vi "Unescape HTTP URL.vi"(1 "escaped string in":string) -> (0 "unescaped string out":string)   [LabVIEW 2017, in "NI_WebServices.lvlib"]
doc: "Replaces escape sequences with the corresponding special characters according to the URL encoding specification RFC 1738."
uses:
  <vilib>/wsapi/NI_WebServices.lvlib
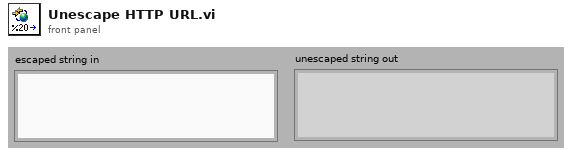
[diagram p1: front panel]
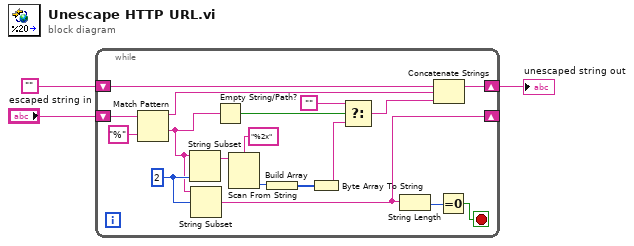
[diagram p0: block diagram]
diagram:
  n1 = while {
    shift-right: [w16] -> _
    shift-left: "escaped string in" -> [w21]
    shift-right: [w18] -> w1
    shift-left: "" -> [w17]
    stop <- w14 stop-if-true
    w19 = 2 ("length (rest)")
    n2 = Match Pattern(string=w21, regular expression="%") -> (before substring=w13:string, after substring=w4:string)  [unwired: 1 in, 2 out]
    n3 = String Subset(string=w4, length (rest)=w19) -> (substring=w10:string)  [unwired: 1 in]
    n4 = String Subset(string=w4, offset (0)=w19) -> (substring=w16:string)  [unwired: 1 in]
    n5 = Empty String/Path?(string/path=w4) -> (empty?=w8:bool)
    n6 = Scan From String(format string="%2x", input string=w10) -> (output 1=w11:u32)  [unwired: 3 in, 3 out]
    n7 = Build Array(w11) -> (w9:u32[])
    n8 = Byte Array To String(unsigned byte array=w9) -> (string=w6:string)
    n9 = Select(t="", s=w8, f=w6) -> (s? t:f=w5:string)
    n10 = String Length(string=w16) -> (length=w15:i32)
    n11 = Concatenate Strings(w17, w13, w5) -> (w18:string)
    n12 = Equal To 0?(x=w15) -> (x = 0?=w14:bool)
  }
  "unescaped string out" <- w1
